vi "Furnace SP calc win.vi"(10 "SP":sgl=10.0 format="%.3f") -> (2 "SP&CRC":u8[](array[numeric]))   [LabVIEW 2011]
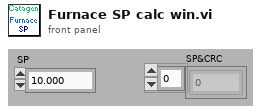
[diagram p1: front panel]
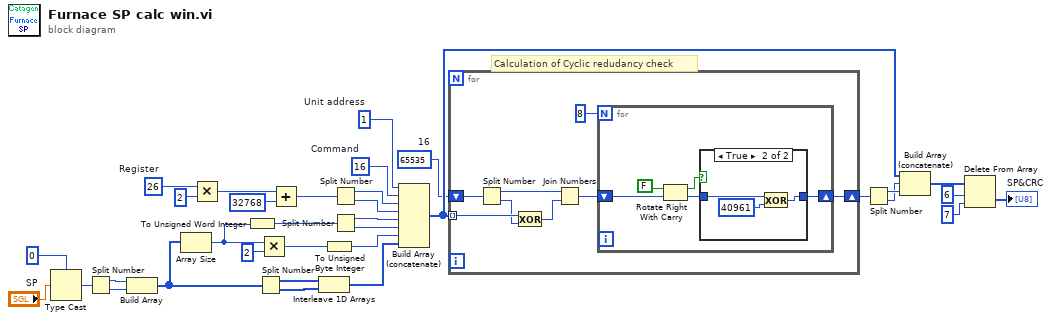
[diagram p0: block diagram]
diagram:
  w8 = u16 26  # Register
  w9 = u8 16  # Command
  w10 = u8 1  # Unit address
  w14 = u16 65535  # 16
  # "Calculation of Cyclic redudancy check"
  n1 = Type Cast(type=0 ("y"), x="SP") -> (*(type *) &x=w2:i32)
  n2 = Split Number(x=w2) -> (hi(x)=w29:u16, lo(x)=w30:u16)
  n3 = Build Array(w29, w30) -> (w28:u16[])
  n4 = Array Size(array=w28) -> (size(s)=w18:i32)
  n5 = Multiply(x=w8, y=u16 2) -> (x*y=w33:u16)
  n6 = To Unsigned Word Integer(number=w18) -> (unsigned 16bit integer=w19:u16)
  n7 = Split Number(x=w28) -> (hi(x)=w27:u8[], lo(x)=w26:u8[])
  n8 = Multiply(x=w18, y=2) -> (x*y=w17:i32)
  n9 = Add(x=w33, y=u16 32768) -> (x+y=w31:u16)
  n10 = Interleave 1D Arrays(w27, w26) -> (w22:u8[])
  n11 = To Unsigned Byte Integer(number=w17) -> (unsigned 8bit integer=w16:u8)
  n12 = Split Number(x=w31) -> (hi(x)=w24:u8, lo(x)=w23:u8)
  n13 = Split Number(x=w19) -> (hi(x)=w21:u8, lo(x)=w20:u8)
  n14 = Build Array (concatenate)(w10, w9, w24, w23, w21, w20, w16, w22) -> (w15:u8[])
  n15 = for {
    tunnel: w15 -> [w42] mode=indexing
    shift-right: [w35] -> w13
    shift-left: w14 -> [w40]
    n16 = Split Number(x=w40) -> (hi(x)=w37:u8, lo(x)=w39:u8)
    n17 = Exclusive Or(1:w39, 2:w42) -> (0:w38:u8)
    n18 = Join Numbers(hi=w37, lo=w38) -> ((hi.lo)=w36:u16)
    n19 = for {
      N: 8 -> [_]
      shift-right: [w43] -> w35
      shift-left: w36 -> [w47]
      n20 = Rotate Right With Carry(2:w47, 3:FALSE ("carry")) -> (0:w44:u16, 1:w45:bool)
      n21 = case shown="True" w45 {
        tunnel: w44 -> [w48 w51]
        tunnel: [w48 w49] -> w43
        frame False {
        }
        frame True {
          n22 = Exclusive Or(1:u16 40961 ("y"), 2:w51) -> (0:w49:u16)
        }
      }
    }
  }
  n23 = Split Number(x=w13) -> (hi(x)=w12:u8, lo(x)=w11:u8)
  n24 = Build Array (concatenate)(w15, w11, w12) -> (w1:u8[])
  n25 = Delete From Array(array=w1, length=6, index=7) -> (deleted portion=→"SP&CRC":u8[])  [unwired: 1 out]
